vi "DI B Fault Clear.vi"(8 "Device Inputs":dbl[](array[numeric]), 10 "B Fault Clear Indexes":T2) -> (3 "B Fault Clear":T1)   [LabVIEW 2016, in "DCM Engine.lvlib"]
uses:
  DCM Engine.lvlib
  <vilib>/Powertrain Controls/Device Drivers/DCM/Tools/FPGA/8 Channels.ctl
  <vilib>/Powertrain Controls/Device Drivers/DCM/Tools/FPGA/DCM - FPGA - Tools.lvlib
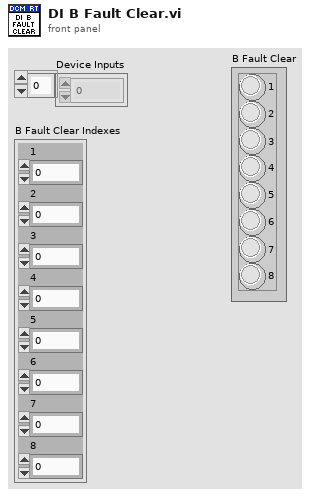
[diagram p1: front panel]
types:
  T1 = typedef "DCM - FPGA - Tools.lvlib/8 Channels.ctl" = cluster{"1":bool, "2":bool, "3":bool, "4":bool, "5":bool, "6":bool, "7":bool, "8":bool}
  T2 = cluster{"1":i32, "2":i32, "3":i32, "4":i32, "5":i32, "6":i32, "7":i32, "8":i32}
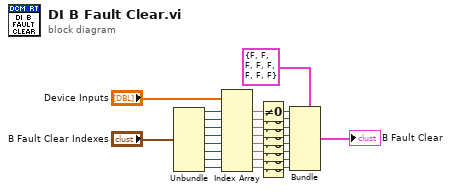
[diagram p0: block diagram]
diagram:
  n1 = Unbundle("B Fault Clear Indexes") -> ("1"=w24:i32, "2"=w17:i32, "3"=w18:i32, "4"=w19:i32, "5"=w20:i32, "6"=w21:i32, "7"=w22:i32, "8"=w23:i32)
  n2 = Index Array(array="Device Inputs", index #1=w24, index #2=w17, index #3=w18, index #4=w19, index #5=w20, index #6=w21, index #7=w22, index #8=w23) -> (element #1=w16:dbl, element #2=w14:dbl, element #3=w13:dbl, element #4=w12:dbl, element #5=w11:dbl, element #6=w10:dbl, element #7=w9:dbl, element #8=w15:dbl)
  n3 = Not Equal To 0?(x=w16) -> (x != 0?=w1:bool)
  n4 = Not Equal To 0?(x=w14) -> (x != 0?=w2:bool)
  n5 = Not Equal To 0?(x=w13) -> (x != 0?=w3:bool)
  n6 = Not Equal To 0?(x=w12) -> (x != 0?=w4:bool)
  n7 = Not Equal To 0?(x=w11) -> (x != 0?=w5:bool)
  n8 = Not Equal To 0?(x=w10) -> (x != 0?=w6:bool)
  n9 = Not Equal To 0?(x=w9) -> (x != 0?=w7:bool)
  n10 = Not Equal To 0?(x=w15) -> (x != 0?=w8:bool)
  n11 = Bundle(cluster=T1 {"1"=FALSE, "2"=FALSE, "3"=FALSE, "4"=FALSE, "5"=FALSE, "6"=FALSE, "7"=FALSE, "8"=FALSE} ("B Fault Clear in"), "1"=w1, "2"=w2, "3"=w3, "4"=w4, "5"=w5, "6"=w6, "7"=w7, "8"=w8) -> (→"B Fault Clear":T1)
